vi "Global DATI MANUALI.vi"() -> ()   [LabVIEW 2019]
panel:
  in  "VIBRAZIONI":T1
  in  "INSERIMENTO VIBRAZIONI?":bool
  in  "DATI MANUALI TRASFORMATORE":T2 caption="INSERIMENTO DATI MANUALI TRASFORMATORE"
  in  "INSERIMENTO DATI MANUALI?":bool
  in  "DATI MANUALI MOTORE DC":cluster{"Vdinamo [V]":dbl} caption="INSERIMENTO DATI MANUALI MOTORE DC"
  in  "DATI MANUALI MOTORE AC":T3 caption="INSERIMENTO DATI MANUALI MOTORE AC"
  in  "DATI MANUALI GENERICO":T4 caption="INSERIMENTO DATI MANUALI GENERICO"
  in  "DATI MANUALI GENERATORE":T5 caption="INSERIMENTO DATI MANUALI GENERATORE"
  in  "DATI MANUALI POMPA":T6 caption="INSERIMENTO DATI MANUALI POMPA"
  # "[mm\\s]"
  # "[ge]"
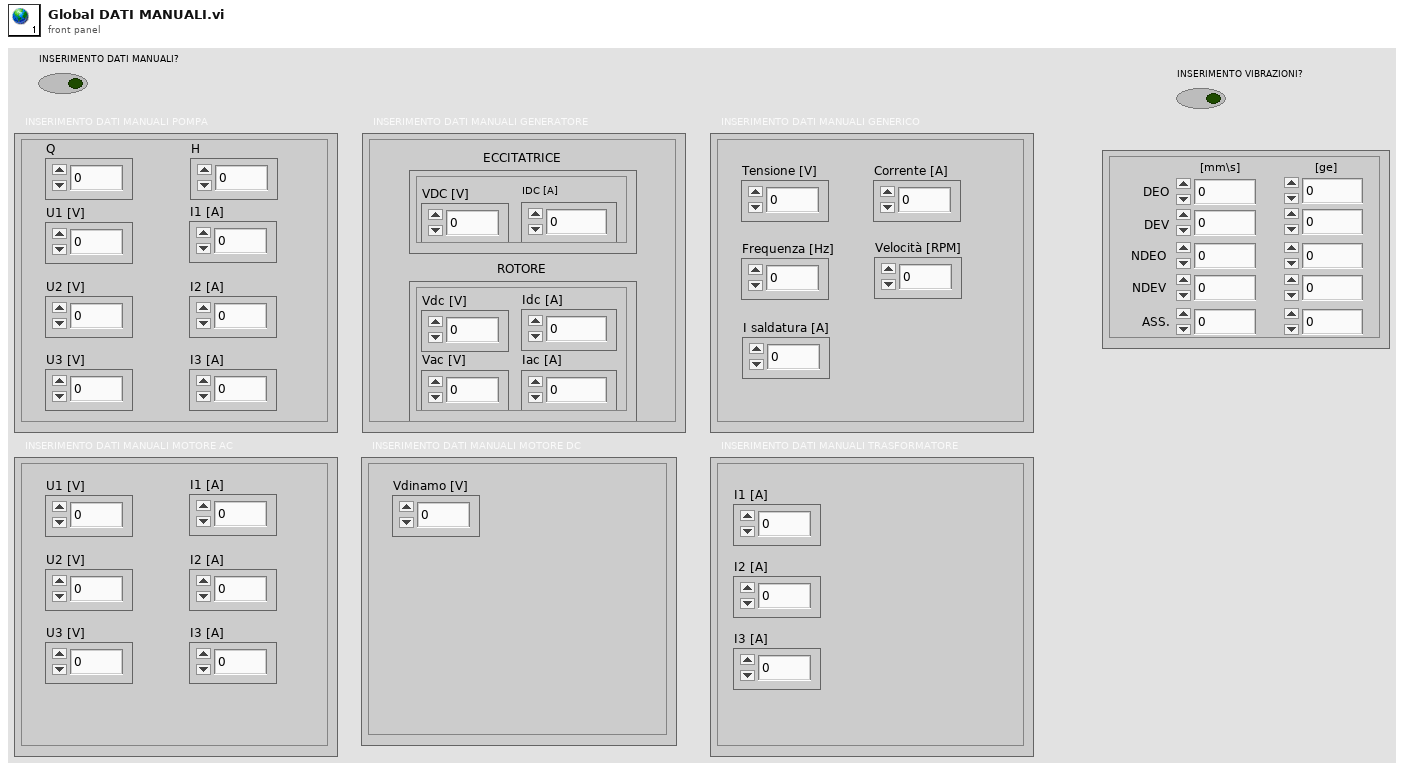
[diagram p1: front panel]
types:
  T1 = cluster{"DEO[mm\\s]":dbl, "DEO[ge]":dbl, "DEV[mm\\s]":dbl, "DEV[ge]":dbl, "NDEO[mm\\s]":dbl, "NDEO[ge]":dbl, "NDEV[mm\\s]":dbl, "NDEV[ge]":dbl, "ASS.[mm\\s]":dbl, "ASS.[ge]":dbl}
  T2 = cluster{"I1 [A]":dbl, "I2 [A]":dbl, "I3 [A]":dbl}
  T3 = cluster{"U1 [V]":dbl, "U2 [V]":dbl, "U3 [V]":dbl, "I1 [A]":dbl, "I2 [A]":dbl, "I3 [A]":dbl}
  T4 = cluster{"Tensione [V]":dbl, "Corrente [A]":dbl, "Frequenza [Hz]":dbl, "Velocità [RPM]":dbl, "I saldatura [A]":dbl}
  T5 = cluster{"ECCITATRICE":cluster{"VDC [V]":dbl, "IDC [A]":dbl}, "ROTORE":cluster{"Vdc [V]":dbl, "Idc [A]":dbl, "Vac [V]":dbl, "Iac [A]":dbl}}
  T6 = cluster{"Q":dbl, "H":dbl, "U1 [V]":dbl, "U2 [V]":dbl, "U3 [V]":dbl, "I1 [A]":dbl, "I2 [A]":dbl, "I3 [A]":dbl}
diagram:
